vi "CAN Read.vi"(8 "error in (no error)":errorcluster, 9 "TimestampBuffer":T2, 11 "Channel":u16) -> (0 "error out":errorcluster, 1 "TimestampBuffer out":T2)   [LabVIEW 2020, in "PCANBasic.lvlib"]
uses:
  <userlib>/PCANBasic/PCANBasic.lvlib
  <userlib>/PCANBasic/ctl/TPCANMsg.ctl
  <userlib>/PCANBasic/PCANBasic.dll
panel:
  out "MessageBuffer out":T1 {"DATA[]" format="%.0x"; "ID" format="%.0x"; "MSGTYPE" format="%.0x"; "DLC" format="%.0x"}
  in  "MessageBuffer":T1 {"DATA[]" format="%.0x"; "ID" format="%.0x"; "MSGTYPE" format="%.0x"; "DLC" format="%.0x"}
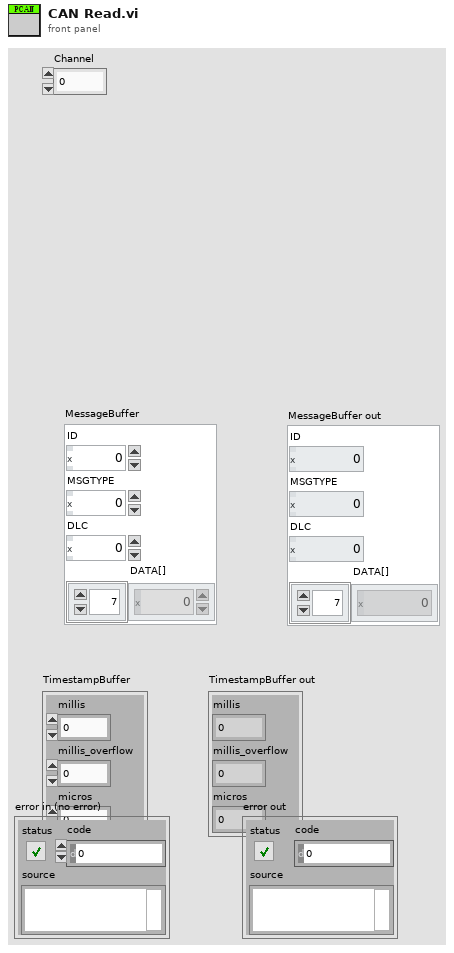
[diagram p1: front panel]
types:
  T1 = typedef "PCANBasic.lvlib/TPCANMsg.ctl" = cluster{"ID":u32, "MSGTYPE":u8, "DLC":u8, "DATA[]":u8[]}
  T2 = cluster{"millis":u32, "millis_overflow":u16, "micros":u16}
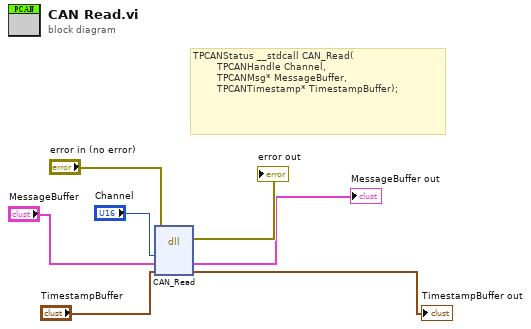
[diagram p0: block diagram]
diagram:
  # "TPCANStatus __stdcall CAN_Read(\n        TPCANHandle Channel, \n        TPCANMsg* MessageBuffer, \n        TPCANTimestamp* TimestampBuffer);"
  n1 = dll-call lib="D:/Program Files (x86)/National Instruments/LabVIEW 2020/user.lib/PCANBasic/PCANBasic.*" fn="CAN_Read"(error in="error in (no error)", "Channel"="Channel", "MessageBuffer", "TimestampBuffer"="TimestampBuffer") -> (error out=→"error out":errorcluster, →"MessageBuffer out":T1, "TimestampBuffer"=→"TimestampBuffer out":T2)  [unwired: 4 in, 1 out]
